vi "Check Status.vi"(8 "error in (no error)":errorcluster, 11 "Collection in":refnum<class "Collection.lvclass">) -> (0 "error out":errorcluster, 1 "Status":string, 2 "Ready?":bool, 3 "Collection out":refnum<class "Collection.lvclass">)   [LabVIEW 2012, in "Collection.lvclass"]
doc: "Checks if the instrument is powered on and updates its member data with the instrument's current status."
uses:
  Collection.lvclass
  Readable/Readable.lvclass
  Collection.lvclass/Collection.ctl
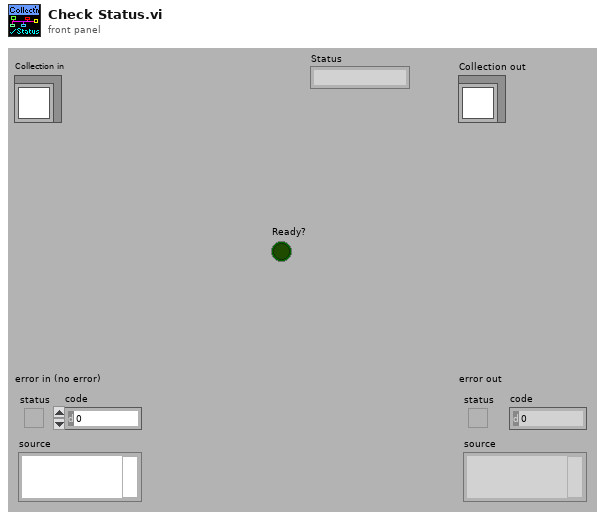
[diagram p1: front panel]
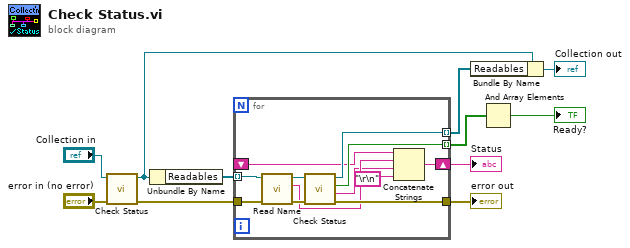
[diagram p0: block diagram]
diagram:
  n1 = call-parent "Check Status.vi"("error in (no error)"="error in (no error)", "Instrument in"="Collection in") -> ("error out"=w9:errorcluster, "Instrument out"=w6:refnum<class "Collection.lvclass">)  [unwired: 8 out]
  n2 = Unbundle By Name(w6) -> ("Readables"=w8:refnum<class "Readable.lvclass">[])
  n3 = for {
    tunnel: w9 -> [w19]
    tunnel: w8 -> [w23] mode=indexing
    tunnel: [w22] -> w7
    tunnel: [w21] -> w4 mode=indexing
    tunnel: [w16] -> w3 mode=indexing
    shift-right: [w15] -> w1
    shift-left: _ -> [w14]
    n4 = call-dynamic "Read Name.vi"("error in (no error)"=w19, "Instrument.lvclass in"=w23) -> ("error out"=w18:errorcluster, "Name"=w17:string, "Instrument.lvclass out"=w20:refnum<class "Readable.lvclass">)  [unwired: 7 out]
    n5 = call-dynamic "Check Status.vi"("error in (no error)"=w18, "Instrument in"=w20) -> ("error out"=w22:errorcluster, "Status"=w13:string, "Ready?"=w16:bool, "Instrument out"=w21:refnum<class "Readable.lvclass">)  [unwired: 6 out]
    n6 = Concatenate Strings(w14, w17, w13, "\r\n") -> (w15:string)
  }
  "error out" <- w7
  "Status" <- w1
  n7 = Bundle By Name(cluster=w6, "Readables"=w4) -> (→"Collection out":refnum<class "Collection.lvclass">)
  n8 = And Array Elements(Boolean array=w3) -> (logical AND=→"Ready?":bool)
